vi "Obsolete_Measure.vi"(8 "error in (no error)":errorcluster, 9 "Variant":variant, 10 "Option":i32, 11 "Avantes in":refnum<class "Avantes.lvclass">) -> (0 "error out":errorcluster, 1 "Data Raw":T1(array[cluster]), 2 "Data":T1(array[cluster]), 3 "Avantes out":refnum<class "Avantes.lvclass">, 4 "Darkspec":T1(array[cluster]), 5 "Time":dbl[](array[numeric]), 6 "Starting Time":dbl)   [LabVIEW 2018]
uses:
  <instrlib>/Classes/CCD/Avantes/Avantes.lvclass
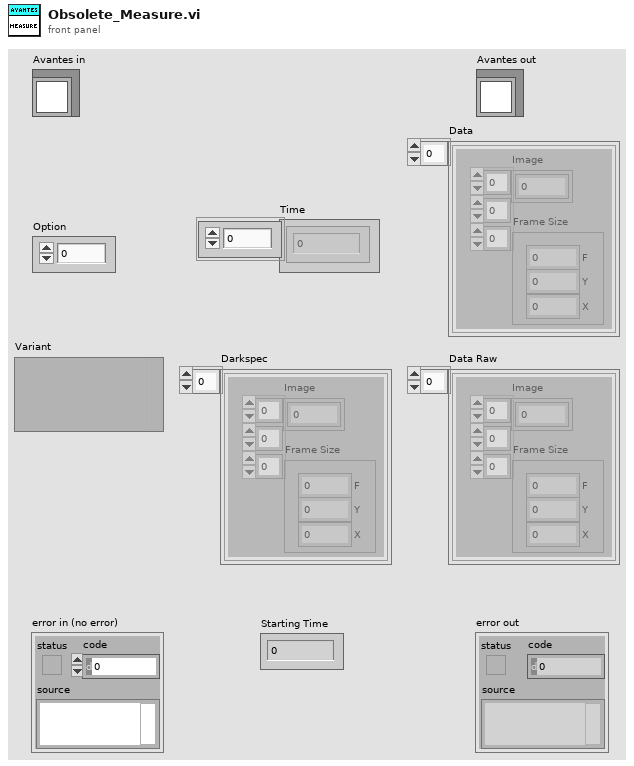
[diagram p1: front panel]
types:
  T1 = cluster{"Image":dbl[][][], "Frame Size":cluster{"F":i32, "Y":i32, "X":i32}}[]
  T2 = cluster{"Frames":i32, "Start Pixel":u16, "Stop Pixel":u16}
  T3 = cluster{"Image":dbl[][][], "Frame Size":cluster{"F":i32, "Y":i32, "X":i32}}
  T4 = typedef "clusterdef.ctl" = cluster{"Len":u16, "ConfigVersion":u16, "UserFriendlyId":u8[], "DetectorType":cluster{"SensorType":u8, "NrPixels":u16, "Fit":sgl[], "NLEnable":u8, "NLCorrect":dbl[], "LowNLCounts":dbl, "HighNLCounts":dbl, "Gain":sgl[], "Reserved":sgl, "Offset":sgl[], "Extern Offset":sgl, "DefectivePixels":u16[]}, "IrradianceType":cluster{"SpectrumCalibrationType":cluster{"SmoothingType":cluster{"m_SmoothPix":u16, "SmoothModel":u8}, "CalInttime":sgl, "CalibConvers":sgl[]}, "CalibrationType":u8, "FiberDiameter":i32}, "SpectrumCalibrationType":cluster{"SmoothingType":cluster{"m_SmoothPix":u16, "SmoothModel":u8}, "CalInttime":sgl, "CalibConvers":sgl[]}, "SpectrumCorrectionType":sgl[], "StandAloneType":cluster{"StandAloneType":u8, "MeasConfigType":cluster{"StartPixel":u16, "StopPixel":u16, "IntegrationTime":sgl, "IntegrationDelay":u32, "NrAverages":u32, "DarkCorrectionType":cluster{"Enable CorDynDark":u8, "ForgetPercentage":u8}, "SmoothingType":cluster{"SmoothPix":u16, "SmoothModel":u8}, "SatDetection":u8, "TriggerType":cluster{"Trigger Mode":u8, "Trigger Source":u8, "Trigger SourceType":u8}, "ControlSettingsType":cluster{"StrobeControl":u16, "LaserDelay":u32, "LaserWidth":u32, "LaserWaveLength":sgl, "StoreToRam":u16}}, "Nmsr":i16}, "DynamicStorageType":cluster{"Nmsr":i32, "Reserved":u8[]}, "TempSensorType":sgl[], "TecControlType":cluster{"Enable":u8, "Setpoint":sgl, "Fit[NR_DAC_POL_COEF]":sgl[]}, "ProcessControlType":cluster{"AnalogLow":sgl[], "AnalogHigh":sgl[], "DigitalLow":sgl[], "DigitalHigh":sgl[]}, "EthernetSettingsType":cluster{"IpAddr":u32, "NetMask":u32, "Gateway":u32, "DhcpEnabled":u8, "TcpPort":u16, "LinkStatus":u8}, "Reserved":u8[], "OemData":u8[]}
  T5 = cluster{"StartPixel":u16, "StopPixel":u16, "IntegrationTime":sgl, "IntegrationDelay":u32, "NrAverages":u32, "DarkCorrectionType":cluster{"Enable CorDynDark":u8, "ForgetPercentage":u8}, "SmoothingType":cluster{"SmoothPix":u16, "SmoothModel":u8}, "SatDetection":u8, "TriggerType":cluster{"Trigger Mode":u8, "Trigger Source":u8, "Trigger SourceType":u8}, "ControlSettingsType":cluster{"StrobeControl":u16, "LaserDelay":u32, "LaserWidth":u32, "LaserWaveLength":sgl, "StoreToRam":u16}}
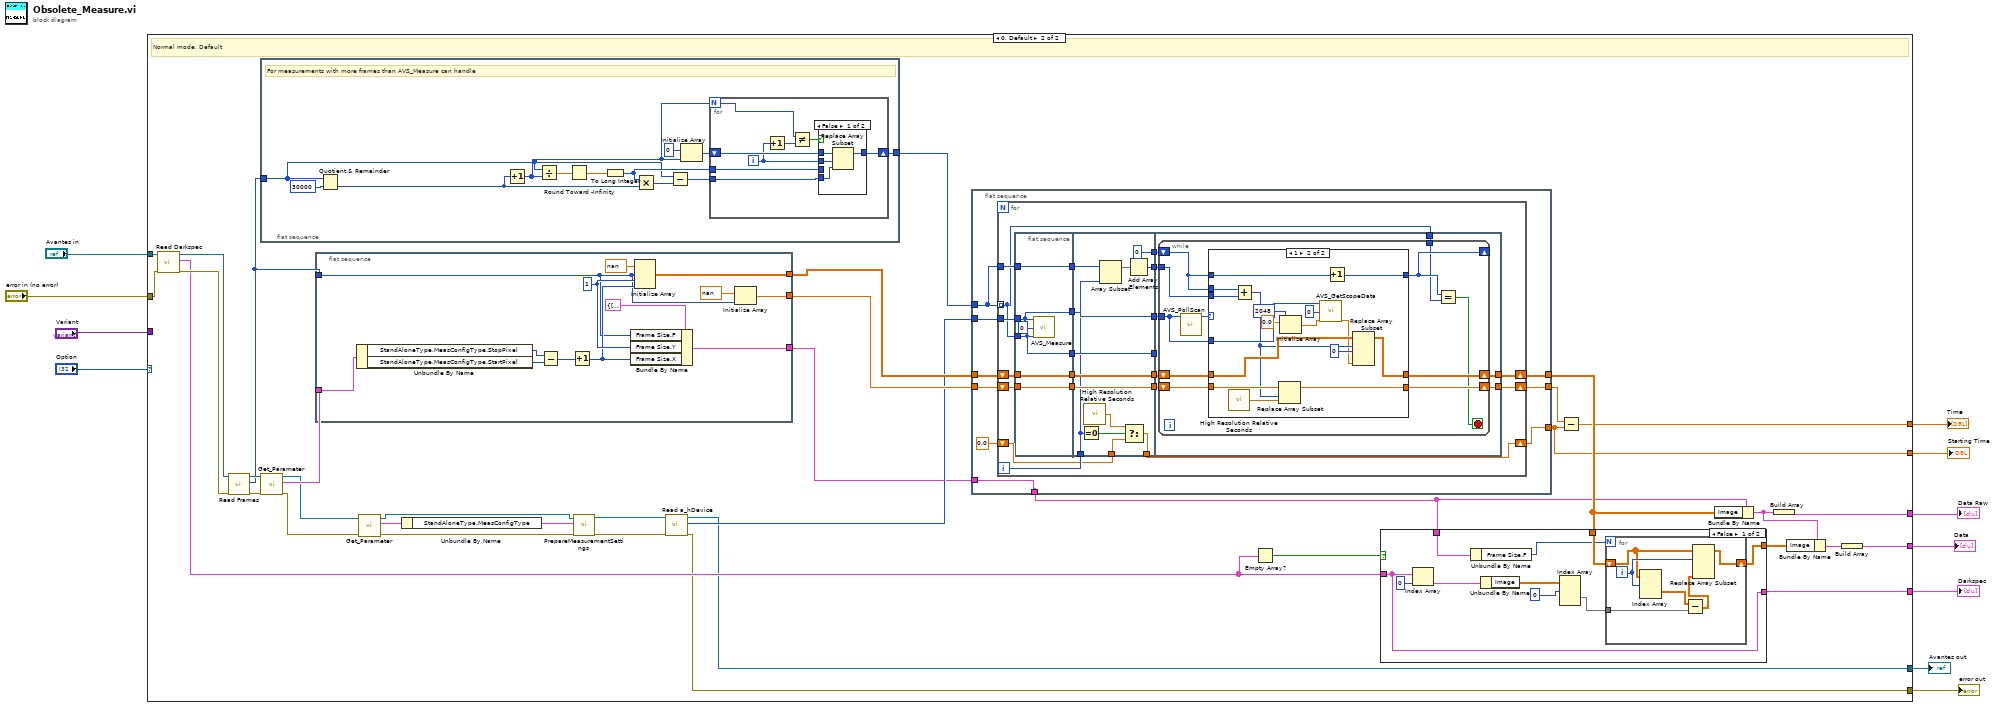
[diagram p0: block diagram]
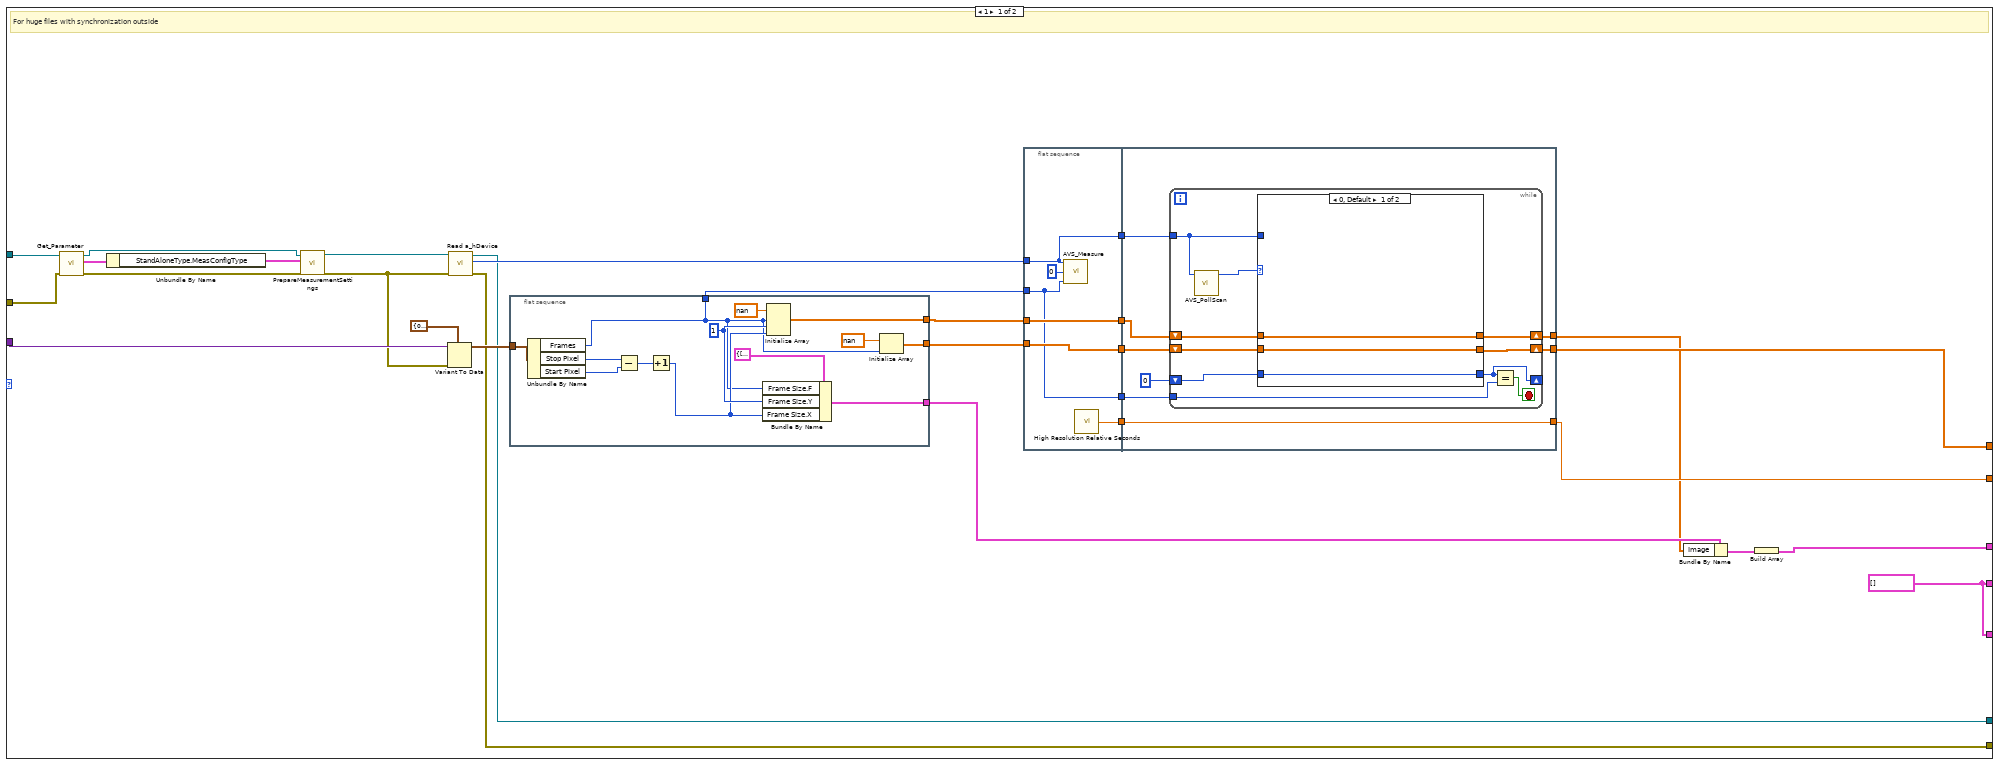
[diagram p2: hidden frame]
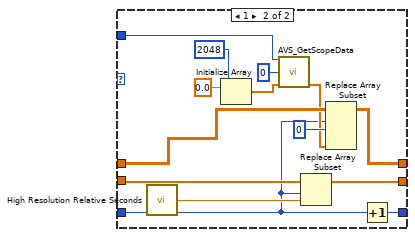
[diagram p3: hidden frame]
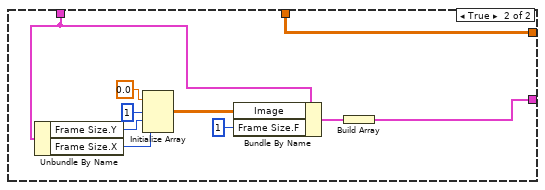
[diagram p4: hidden frame]
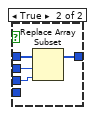
[diagram p6: hidden frame]
diagram:
  n1 = case shown="0, Default" "Option" {
    tunnel: "Avantes in" -> [w15 w130]
    tunnel: "error in (no error)" -> [w14 w129]
    tunnel: [w28 w101] -> w9
    tunnel: [w29 w100] -> w8
    tunnel: [w25 w99] -> w7
    tunnel: [w25 w98] -> w6
    tunnel: [w21 w97] -> w5
    tunnel: [w26 w96] -> w4
    tunnel: [w27 w95] -> w3
    tunnel: "Variant" -> [w40 _]
    frame 1 {
      w25 = T1 []
      # "For huge files with synchronization outside"
      n2 = call-dynamic "Get_Parameter.vi"("error in (no error)"=w14, "Avantes in"=w15) -> ("error out"=w16:errorcluster, "DeviceConfig"=w19:T4, "Avantes out"=w17:refnum<class "Avantes.lvclass">)  [unwired: 7 in]
      n3 = Unbundle By Name(w19) -> ("StandAloneType.MeasConfigType"=w18:T5)
      n4 = call-dynamic "PrepareMeasurementSettings.vi"("error in (no error)"=w16, "MeasConfigType"=w18, "Avantes in"=w17) -> ("error out"=w12:errorcluster, "Avantes out"=w13:refnum<class "Avantes.lvclass">)  [unwired: 7 in]
      n5 = Variant To Data(error in=w12, type=T2 {"Frames"=0, "Start Pixel"=0, "Stop Pixel"=0}, Variant=w40) -> (data=w38:T2)  [unwired: 1 out]
      n6 = call-dynamic "Read a_hDevice.vi"("error in (no error)"=w12, "Avantes in"=w13) -> ("error out"=w27:errorcluster, "a_hDevice"=w37:i32, "Avantes out"=w26:refnum<class "Avantes.lvclass">)  [unwired: 7 in]
      n7 = flat-sequence {
        tunnel: [w91] -> w24
        tunnel: [w90] -> w33
        tunnel: [w88] -> w32
        tunnel: w38 -> [w87]
        tunnel: [w82] -> w36
        frame #0 {
          w92 = 1 ("Frame Size.Y")
          n8 = Unbundle By Name(w87) -> ("Frames"=w82:i32, "Stop Pixel"=w86:u16, "Start Pixel"=w85:u16)
          n9 = Subtract(x=w86, y=w85) -> (x-y=w84:u16)
          n10 = Increment(x=w84) -> (x+1=w83:u16)
          n11 = Bundle By Name(cluster=T3 {"Image"=[], "Frame Size"={"F"=0, "Y"=0, "X"=0}} ("Cluster"), "Frame Size.F"=w82, "Frame Size.Y"=w92, "Frame Size.X"=w83) -> (w91:T3)
          n12 = Initialize Array(nan ("element"), w82, w92, w83) -> (w90:dbl[][][])
          n13 = Initialize Array(nan ("element"), w82) -> (w88:dbl[])
        }
      }
      n14 = flat-sequence {
        tunnel: w37 -> [w45]
        tunnel: w36 -> [w41]
        tunnel: [w45] -> w35
        tunnel: [w44] -> w34
        tunnel: w33 -> [w44]
        tunnel: w32 -> [w43]
        tunnel: [w43] -> w31
        tunnel: [w42] -> w30
        tunnel: [w41] -> w20
        tunnel: w35 -> [w53]
        tunnel: w34 -> [w52]
        tunnel: w31 -> [w51]
        tunnel: [w50] -> w23
        tunnel: [w49] -> w28
        tunnel: w30 -> [w48]
        tunnel: [w48] -> w29
        tunnel: w20 -> [w47]
        frame #0 {
          n15 = call <instrlib>:"AVS_Measure.vi"("a_hDevice"=w45, "a_hWnd"=0, "a_Nmsr"=w41) -> ()  [unwired: 12 in, 1 out]
          n16 = call <vilib>:"High Resolution Relative Seconds.vi"() -> ("relative seconds"=w42:dbl)
        }
        frame #1 {
          n17 = while {
            shift-right: [w62] -> w49
            shift-left: w51 -> [w63]
            shift-right: [w60] -> w50
            shift-left: w52 -> [w61]
            shift-right: [w57] -> _
            shift-left: 0 -> [w59]
            tunnel: w53 -> [w56]
            tunnel: w47 -> [w55]
            stop <- w58 stop-if-true
            n18 = call <instrlib>:"AVS_PollScan.vi"("a_hDevice"=w56) -> ("Output Value"=w64:i32)  [unwired: 8 in]
            n19 = case shown="0, Default" w64 {
              tunnel: w63 -> [w67 w80]
              tunnel: [w67 w78] -> w62
              tunnel: w61 -> [w65 w77]
              tunnel: [w65 w75] -> w60
              tunnel: w59 -> [w66 w69]
              tunnel: [w66 w74] -> w57
              tunnel: w56 -> [_ w68]
              frame 0, Default {
              }
              frame 1 {
                n20 = call <vilib>:"High Resolution Relative Seconds.vi"() -> ("relative seconds"=w79:dbl)
                n21 = Initialize Array(0.0 ("element"), 2048 ("dimension size")) -> (w73:dbl[])
                n22 = call <instrlib>:"AVS_GetScopeData.vi"("a_hDevice"=w68, "a_pTimeLabel"=u32 0, "a_pSpectrum"=w73) -> ("a_pSpectrum"=w70:dbl[])  [unwired: 10 in, 2 out]
                n23 = Replace Array Subset(array=w80, new element=w79, index=w69) -> (w78:dbl[])
                n24 = Replace Array Subset(array=w77, new element=w70, index (dim 0)=w69, index (dim 1)=0 ("disabled index (row)")) -> (w75:dbl[][][])  [unwired: 1 in]
                n25 = Increment(x=w69) -> (x+1=w74:i32)
              }
            }
            n26 = Equal?(x=w57, y=w55) -> (x = y?=w58:bool)
          }
        }
      }
      n27 = Bundle By Name(cluster=w24, "Image"=w23) -> (w22:T3)
      n28 = Build Array(w22) -> (w21:T1)
    }
    frame 0, Default {
      # "Normal mode, Default"
      n29 = call-dynamic "Read Darkspec.vi"("error in (no error)"=w129, "Avantes in"=w130) -> ("error out"=w127:errorcluster, "Darkspec"=w119:T1, "Avantes out"=w128:refnum<class "Avantes.lvclass">)  [unwired: 7 in]
      n30 = call-dynamic "Read Frames.vi"("error in (no error)"=w127, "Avantes in"=w128) -> ("error out"=w125:errorcluster, "Frames"=w123:i32, "Avantes out"=w126:refnum<class "Avantes.lvclass">)  [unwired: 7 in]
      n31 = flat-sequence {
        tunnel: w123 -> [w259]
        tunnel: [w258] -> w122
        frame #0 {
          # "For measurements with more frames than AVS_Measure can handle"
          n32 = Quotient & Remainder(x=w259, y=30000) -> (floor(x/y)=w263:i32)  [unwired: 1 out]
          n33 = Increment(x=w263) -> (x+1=w264:i32)
          n34 = Divide(x=w259, y=w264) -> (x/y=w268:dbl)
          n35 = Round Toward -Infinity(1:w268) -> (0:w265:dbl)
          n36 = To Long Integer(number=w265) -> (32bit integer=w261:i32)
          n37 = Multiply(x=w261, y=w263) -> (x*y=w262:i32)
          n38 = Subtract(x=w259, y=w262) -> (x-y=w260:i32)
          n39 = Initialize Array(0, w264) -> (w266:i32[])
          n40 = for {
            N: w264 -> [w276]
            shift-right: [w271] -> w258
            shift-left: w266 -> [w274]
            tunnel: w261 -> [w272]
            tunnel: w260 -> [w270]
            i -> [w273]
            n41 = Increment(x=w273) -> (x+1=w277:i32)
            n42 = Not Equal?(x=w276, y=w277) -> (x != y?=w275:bool)
            n43 = case shown="False" w275 {
              tunnel: w274 -> [w281 w285]
              tunnel: w273 -> [w280 w284]
              tunnel: w272 -> [_ w283]
              tunnel: [w278 w282] -> w271
              tunnel: w270 -> [w279 _]
              frame False {
                n44 = Replace Array Subset(array=w281, new element=w279, index=w280) -> (w278:i32[])
              }
              frame True {
                n45 = Replace Array Subset(array=w285, new element=w283, index=w284) -> (w282:i32[])
              }
            }
          }
        }
      }
      n46 = call-dynamic "Get_Parameter.vi"("error in (no error)"=w125, "Avantes in"=w126) -> ("error out"=w111:errorcluster, "DeviceConfig"=w124:T4, "Avantes out"=w112:refnum<class "Avantes.lvclass">)  [unwired: 7 in]
      n47 = flat-sequence {
        tunnel: w124 -> [w256]
        tunnel: w123 -> [w246]
        tunnel: [w249] -> w103
        tunnel: [w248] -> w121
        tunnel: [w245] -> w120
        frame #0 {
          w251 = 1 ("Frame Size.Y")
          n48 = Unbundle By Name(w256) -> ("StandAloneType.MeasConfigType.StopPixel"=w255:u16, "StandAloneType.MeasConfigType.StartPixel"=w254:u16)
          n49 = Subtract(x=w255, y=w254) -> (x-y=w253:u16)
          n50 = Increment(x=w253) -> (x+1=w250:u16)
          n51 = Bundle By Name(cluster=T3 {"Image"=[], "Frame Size"={"F"=0, "Y"=0, "X"=0}} ("Cluster"), "Frame Size.F"=w246, "Frame Size.Y"=w251, "Frame Size.X"=w250) -> (w249:T3)
          n52 = Initialize Array(nan ("element"), w246, w251, w250) -> (w248:dbl[][][])
          n53 = Initialize Array(nan ("element"), w246) -> (w245:dbl[])
        }
      }
      n54 = call-dynamic "Get_Parameter.vi"("error in (no error)"=w111, "Avantes in"=w112) -> ("error out"=w107:errorcluster, "DeviceConfig"=w110:T4, "Avantes out"=w108:refnum<class "Avantes.lvclass">)  [unwired: 7 in]
      n55 = Unbundle By Name(w110) -> ("StandAloneType.MeasConfigType"=w109:T5)
      n56 = call-dynamic "PrepareMeasurementSettings.vi"("error in (no error)"=w107, "MeasConfigType"=w109, "Avantes in"=w108) -> ("error out"=w106:errorcluster, "Avantes out"=w105:refnum<class "Avantes.lvclass">)  [unwired: 7 in]
      n57 = call-dynamic "Read a_hDevice.vi"("error in (no error)"=w106, "Avantes in"=w105) -> ("error out"=w95:errorcluster, "a_hDevice"=w113:i32, "Avantes out"=w96:refnum<class "Avantes.lvclass">)  [unwired: 7 in]
      n58 = flat-sequence {
        tunnel: w122 -> [w161]
        tunnel: w113 -> [w165]
        tunnel: w121 -> [w163]
        tunnel: w120 -> [w162]
        tunnel: [w160] -> w117
        tunnel: [w159] -> w104
        tunnel: [w158] -> w100
        tunnel: [w157] -> w102
        tunnel: w103 -> [w157]
        frame #0 {
          n59 = for {
            tunnel: w161 -> [w168] mode=indexing
            tunnel: w165 -> [w186]
            shift-right: [w183] -> w158
            shift-left: 0.0 ("relative seconds") -> [w184]
            shift-right: [w167] -> w160
            shift-left: w163 -> [w178]
            shift-right: [w166] -> w159
            shift-left: w162 -> [w175]
            tunnel: w161 -> [w172]
            i -> [w185]
            n60 = flat-sequence {
              tunnel: w186 -> [w191]
              tunnel: w168 -> [w190]
              tunnel: [w191] -> w182
              tunnel: [w190] -> w180
              tunnel: w178 -> [w189]
              tunnel: [w189] -> w176
              tunnel: w175 -> [w188]
              tunnel: [w188] -> w173
              tunnel: w172 -> [w187]
              tunnel: [w187] -> w171
              tunnel: w185 -> [w193]
              tunnel: w184 -> [w203]
              tunnel: [w202] -> w183
              tunnel: w182 -> [w201]
              tunnel: [w201] -> w181
              tunnel: w180 -> [w200]
              tunnel: [w200] -> w179
              tunnel: [w199] -> w177
              tunnel: w176 -> [w199]
              tunnel: [w198] -> w174
              tunnel: w173 -> [w198]
              tunnel: w171 -> [w197]
              tunnel: [w195] -> w170
              tunnel: [0] -> w169
              tunnel: w181 -> [w213]
              tunnel: w179 -> [_]
              tunnel: w177 -> [w211]
              tunnel: w174 -> [w212]
              tunnel: w170 -> [w210]
              tunnel: w169 -> [w209]
              tunnel: w168 -> [w208]
              tunnel: [w207] -> w167
              tunnel: [w206] -> w166
              frame #0 {
                n61 = call <instrlib>:"AVS_Measure.vi"("a_hDevice"=w191, "a_hWnd"=0, "a_Nmsr"=w190) -> ()  [unwired: 12 in, 1 out]
              }
              frame #1 {
                n62 = Equal To 0?(x=w193) -> (x = 0?=w205:bool)
                n63 = call <vilib>:"High Resolution Relative Seconds.vi"() -> ("relative seconds"=w204:dbl)
                n64 = Array Subset(array=w197, length=w193) -> (w196:i32[])  [unwired: 1 in]
                n65 = Select(t=w204, s=w205, f=w203) -> (s? t:f=w202:dbl)
                n66 = Add Array Elements(numeric array=w196) -> (sum=w195:i32)
              }
              frame #2 {
                n67 = while {
                  tunnel: w213 -> [w223]
                  shift-right: [w220] -> w206
                  shift-left: w212 -> [w221]
                  shift-right: [w218] -> w207
                  shift-left: w211 -> [w219]
                  tunnel: w210 -> [w222]
                  shift-right: [w216] -> _
                  shift-left: w209 -> [w217]
                  tunnel: w208 -> [w215]
                  stop <- w214 stop-if-true
                  n68 = call <instrlib>:"AVS_PollScan.vi"("a_hDevice"=w223) -> ("Output Value"=w224:i32)  [unwired: 8 in]
                  n69 = case shown="1" w224 {
                    tunnel: w223 -> [_ w244]
                    tunnel: w222 -> [_ w235]
                    tunnel: w221 -> [w227 w242]
                    tunnel: [w227 w240] -> w220
                    tunnel: w219 -> [w225 w239]
                    tunnel: [w225 w236] -> w218
                    tunnel: w217 -> [_ w234]
                    tunnel: w217 -> [w226 w233]
                    tunnel: [w226 w232] -> w216
                    frame 0, Default {
                    }
                    frame 1 {
                      n70 = call <vilib>:"High Resolution Relative Seconds.vi"() -> ("relative seconds"=w241:dbl)
                      n71 = Add(x=w234, y=w235) -> (x+y=w238:i32)
                      n72 = Replace Array Subset(array=w242, new element=w241, index=w238) -> (w240:dbl[])
                      n73 = Initialize Array(0.0 ("element"), 2048 ("dimension size")) -> (w231:dbl[])
                      n74 = call <instrlib>:"AVS_GetScopeData.vi"("a_hDevice"=w244, "a_pTimeLabel"=u32 0, "a_pSpectrum"=w231) -> ("a_pSpectrum"=w228:dbl[])  [unwired: 10 in, 2 out]
                      n75 = Increment(x=w233) -> (x+1=w232:i32)
                      n76 = Replace Array Subset(array=w239, new element=w228, index (dim 0)=w238, index (dim 1)=0 ("disabled index (row)")) -> (w236:dbl[][][])  [unwired: 1 in]
                    }
                  }
                  n77 = Equal?(x=w216, y=w215) -> (x = y?=w214:bool)
                }
              }
            }
          }
        }
      }
      n78 = Empty Array?(array=w119) -> (empty?=w118:bool)
      n79 = case shown="False" w118 {
        tunnel: w119 -> [w137 _]
        tunnel: [w137 w149] -> w99
        tunnel: w102 -> [w132 w147]
        tunnel: w117 -> [w139 w148]
        tunnel: [w133 w148] -> w115
        frame False {
          n80 = Index Array(array=w137, index=0) -> (element=w138:T3)
          n81 = Unbundle By Name(w132) -> ("Frame Size.F"=w131:i32)
          n82 = Unbundle By Name(w138) -> ("Image"=w136:dbl[][][])
          n83 = Index Array(array=w136, index (dim 0)=0 ("index")) -> (element=w134:dbl[][])  [unwired: 2 in]
          n84 = for {
            N: w131 -> [_]
            shift-right: [w141] -> w133
            shift-left: w139 -> [w145]
            tunnel: w134 -> [w143]
            i -> [w146]
            n85 = Index Array(array=w145, index (dim 0)=w146) -> (element=w144:dbl[][])  [unwired: 2 in]
            n86 = Subtract(x=w144, y=w143) -> (x-y=w142:dbl[][])
            n87 = Replace Array Subset(array=w145, new element=w142, index (dim 0)=w146) -> (w141:dbl[][][])  [unwired: 2 in]
          }
        }
        frame True {
          n88 = Unbundle By Name(w147) -> ("Frame Size.Y"=w155:i32, "Frame Size.X"=w154:i32)
          n89 = Initialize Array(0.0 ("element"), 1 ("dimension size"), w155, w154) -> (w151:dbl[][][])
          n90 = Bundle By Name(cluster=w147, "Image"=w151, "Frame Size.F"=1) -> (w150:T3)
          n91 = Build Array(w150) -> (w149:T1)
        }
      }
      n92 = Subtract(x=w104, y=w100) -> (x-y=w101:dbl[])
      n93 = Bundle By Name(cluster=w102, "Image"=w117) -> (w116:T3)
      n94 = Build Array(w116) -> (w97:T1)
      n95 = Bundle By Name(cluster=w116, "Image"=w115) -> (w114:T3)
      n96 = Build Array(w114) -> (w98:T1)
    }
  }
  "Time" <- w9
  "Starting Time" <- w8
  "Data Raw" <- w5
  "Data" <- w6
  "Darkspec" <- w7
  "error out" <- w3
  "Avantes out" <- w4
